vi "DDS9959 Send.vi"(8 "error in (no error)":errorcluster, 9 "Output Array":string[](array[string]), 10 "USB Out Endpoint":i16, 11 "VISA resource name":refnum<visa-resource-name>) -> (0 "error out":errorcluster, 3 "VISA resource name":refnum<visa-resource-name>)   [LabVIEW 2012]
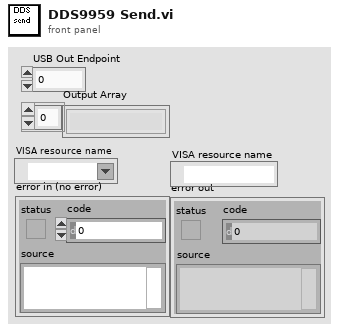
[diagram p1: front panel]
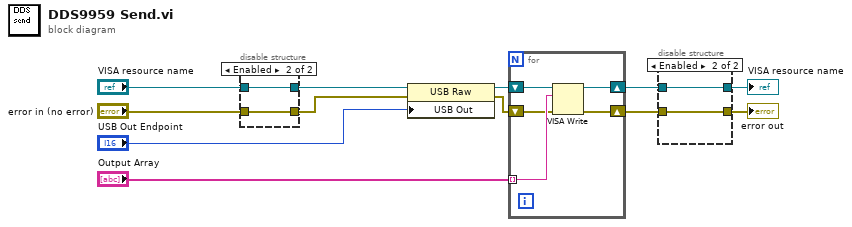
[diagram p0: block diagram]
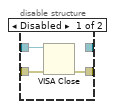
[diagram p2: hidden frame]
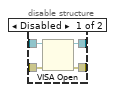
[diagram p3: hidden frame]
diagram:
  n1 = disable-structure shown="Enabled" {
    disable-tunnel: "error in (no error)" -> [w16 w17]
    disable-tunnel: "VISA resource name" -> [w15 w18]
    disable-tunnel: [w14 w18] -> w6
    disable-tunnel: [w13 w17] -> w5
    frame Disabled {
      n2 = VISA Open(error in (no error)=w16, VISA resource name=w15) -> (VISA resource name=w14:refnum<visa-resource-name>, error out=w13:errorcluster)  [unwired: 3 in]
    }
    frame Enabled {
    }
  }
  n3 = property class="USB Raw"(reference=w6, error in=w5, "USB Out"="USB Out Endpoint") -> (reference out=w12:refnum<visa-resource-name>, error out=w11:errorcluster)
  n4 = for {
    shift-right: [w23] -> w2
    shift-left: w12 -> [w19]
    shift-right: [w22] -> w4
    shift-left: w11 -> [w20]
    tunnel: "Output Array" -> [w21] mode=indexing
    n5 = VISA Write(VISA resource name=w19, write buffer=w21, error in (no error)=w20) -> (VISA resource name out=w23:refnum<visa-resource-name>, error out=w22:errorcluster)  [unwired: 1 out]
  }
  n6 = disable-structure shown="Enabled" {
    disable-tunnel: w4 -> [w26 w28]
    disable-tunnel: w2 -> [w25 w27]
    disable-tunnel: [w24 w28] -> w3
    disable-tunnel: [_ w27] -> w1
    frame Disabled {
      n7 = VISA Close(VISA resource name=w25, error in (no error)=w26) -> (error out=w24:errorcluster)
    }
    frame Enabled {
    }
  }
  "error out" <- w3
  "VISA resource name" <- w1
